vi "I32Notifier Get.vi"(8 "error in (no error)":errorcluster, 11 "I32Notifier in":refnum<class "I32Notifier.lvclass">) -> (0 "error out":errorcluster, 2 "LastValue":i32, 3 "I32Notifier out":refnum<class "I32Notifier.lvclass">)   [LabVIEW 2018, in "I32Notifier.lvclass"]
uses:
  I32Notifier.lvclass
  I32Notifier.lvclass/I32Notifier.ctl
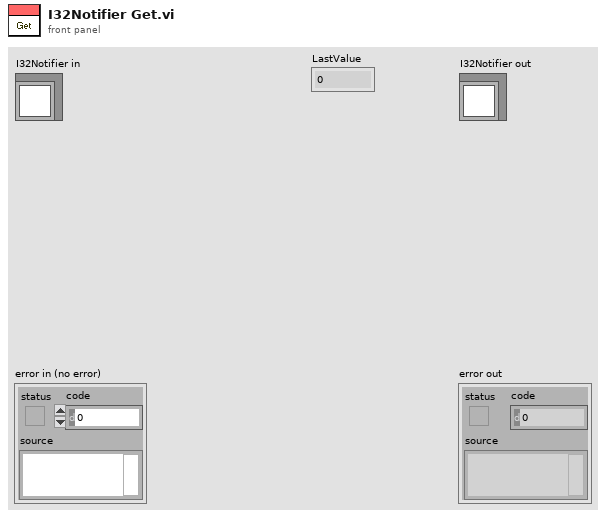
[diagram p1: front panel]
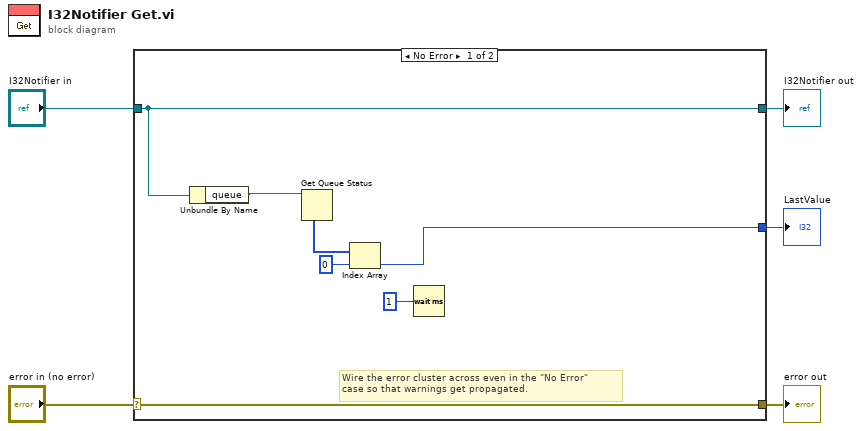
[diagram p0: block diagram]
diagram:
  n1 = case shown="No Error" "error in (no error)" {
    selector: "error in (no error)" -> [w12 w14]
    tunnel: [w12 w14] -> w4
    tunnel: [w11 w13] -> w2
    tunnel: "I32Notifier in" -> [w11 w13]
    tunnel: [w8 _] -> w1
    frame No Error {
      # "Wire the error cluster across even in the \"No Error\"\ncase so that warnings get propagated."
      n2 = Unbundle By Name(w11) -> ("queue"=w10:refnum<queue>)
      n3 = Get Queue Status(queue=w10) -> (elements=w9:i32[])  [unwired: 2 in, 7 out]
      n4 = Index Array(array=w9, index=0) -> (element=w8:i32)
      n5 = Wait (ms)(milliseconds to wait=u32 1) -> ()  [unwired: 1 out]
    }
    frame Error {
    }
  }
  "error out" <- w4
  "I32Notifier out" <- w2
  "LastValue" <- w1
